vi "MoveDashboard.vi"(11 "VI in":refnum<vi>) -> ()   [LabVIEW 2014]
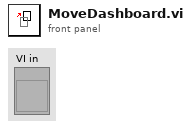
[diagram p1: front panel]
types:
  T1 = typedef "LVAllMonitorsDisplayTypeDef.ctl" = cluster{"Bounds":cluster{"Left":i16, "Top":i16, "Right":i16, "Bottom":i16}, "Depth":i16}[]
  T2 = typedef "LVRectTypeDef.ctl" = cluster{"Left":i16, "Top":i16, "Right":i16, "Bottom":i16}
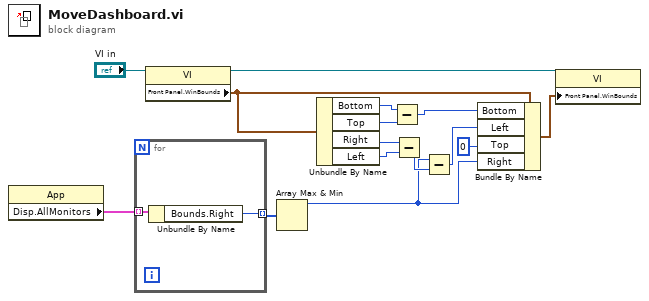
[diagram p0: block diagram]
diagram:
  n1 = property class="App"() -> ("Disp.AllMonitors"=w11:T1)  [unwired: 2 in, 2 out]
  n2 = for {
    tunnel: w11 -> [w17] mode=indexing
    tunnel: [w16] -> w10 mode=indexing
    n3 = Unbundle By Name(w17) -> ("Bounds.Right"=w16:i16)
  }
  n4 = property class="VI"(reference="VI in") -> (reference out=w14:refnum<vi>, "Front Panel.WinBounds"=w9:T2)  [unwired: 1 in, 1 out]
  n5 = Array Max & Min(array=w10) -> (max value=w2:i16)  [unwired: 3 out]
  n6 = Unbundle By Name(w9) -> ("Bottom"=w7:i16, "Top"=w8:i16, "Right"=w5:i16, "Left"=w4:i16)
  n7 = Subtract(x=w7, y=w8) -> (x-y=w6:i16)
  n8 = Subtract(x=w5, y=w4) -> (x-y=w3:i16)
  n9 = Subtract(x=w2, y=w3) -> (x-y=w1:i16)
  n10 = Bundle By Name(cluster=w9, "Bottom"=w6, "Left"=w1, "Top"=i16 0, "Right"=w2) -> (w13:T2)
  n11 = property class="VI"(reference=w14, "Front Panel.WinBounds"=w13) -> ()  [unwired: 1 in, 2 out]
